vi "Main.vi"(6 "Action":T1, 8 "error in":errorcluster, 11 "Data In":variant) -> (0 "error out":errorcluster, 3 "Data out":T2)   [LabVIEW 2015, in "App Info.lvlib"]
doc: "Main VI of App Info LV2."
uses:
  App Info.lvlib
  Core Data.ctl
  Action.ctl
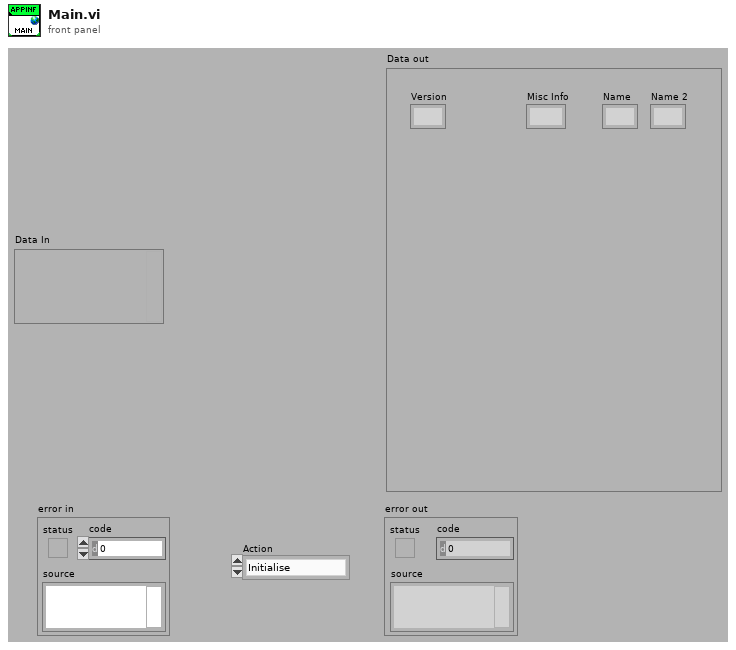
[diagram p1: front panel]
types:
  T1 = typedef "App Info.lvlib/Action.ctl" = enum16{"Initialise", "get All", "set Version", "set Misc Info", "set Name", "set Name 2"}
  T2 = typedef "App Info.lvlib/Core Data.ctl" = cluster{"Version":string, "Misc Info":string, "Name":string, "Name 2":string}
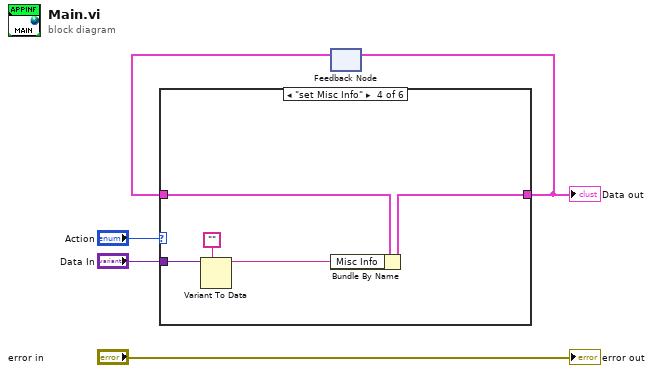
[diagram p0: block diagram]
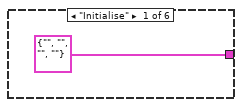
[diagram p2: hidden frame]
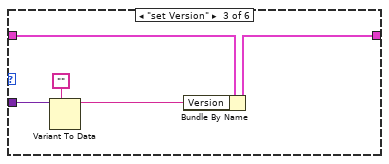
[diagram p4: hidden frame]
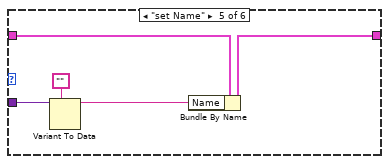
[diagram p5: hidden frame]
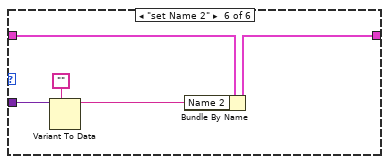
[diagram p6: hidden frame]
diagram:
  n1 = feedback #1() -> (w3:T2)  [unwired: 1 in]
  n2 = case shown="\"set Misc Info\"" "Action" {
    tunnel: [T2 {"Version"="", "Misc Info"="", "Name"="", "Name 2"=""} ("Data in") w7 w8 w13 w18 w23] -> w4
    tunnel: w3 -> [_ w7 w10 w15 w20 w25]
    tunnel: "Data In" -> [_ _ w12 w17 w22 w27]
    frame "Initialise" {
    }
    frame "get All" {
    }
    frame "set Version" {
      n3 = Variant To Data(type="", Variant=w12) -> (data=w9:string)  [unwired: 1 in, 1 out]
      n4 = Bundle By Name(cluster=w10, "Version"=w9) -> (w8:T2)
    }
    frame "set Misc Info" {
      n5 = Variant To Data(type="", Variant=w17) -> (data=w14:string)  [unwired: 1 in, 1 out]
      n6 = Bundle By Name(cluster=w15, "Misc Info"=w14) -> (w13:T2)
    }
    frame "set Name" {
      n7 = Variant To Data(type="", Variant=w22) -> (data=w19:string)  [unwired: 1 in, 1 out]
      n8 = Bundle By Name(cluster=w20, "Name"=w19) -> (w18:T2)
    }
    frame "set Name 2" {
      n9 = Variant To Data(type="", Variant=w27) -> (data=w24:string)  [unwired: 1 in, 1 out]
      n10 = Bundle By Name(cluster=w25, "Name 2"=w24) -> (w23:T2)
    }
  }
  "Data out" <- w4
  n11 = feedback-in #1(w4) -> ()
  "error out" <- "error in"
